vi "niRFUtil FTW Compute AAF Parameter.vi"(10 "Stopband Attenuation (dB)":dbl=85.0 format="%.2f", 11 "Decimation Rate":dbl=1.0) -> (2 "Kaiser Beta":dbl format="%.2f", 3 "AAF Order":i32)   [LabVIEW 2015, in "niRFUtil.lvlib"]
uses:
  niRFUtil.lvlib
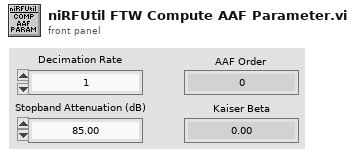
[diagram p1: front panel]
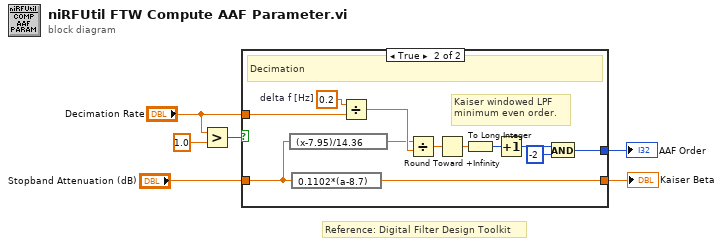
[diagram p0: block diagram]
diagram:
  # "Reference: Digital Filter Design Toolkit"
  n1 = Greater?(x="Decimation Rate", y=1.0) -> (0:w5:bool)
  n2 = case shown="True" w5 {
    tunnel: "Decimation Rate" -> [_ w10]
    tunnel: [_ w9] -> w3
    tunnel: [_ w8] -> w2
    tunnel: "Stopband Attenuation (dB)" -> [_ w7]
    frame False {
    }
    frame True {
      w11 = 0.2  # delta f [Hz]
      # "Kaiser windowed LPF\nminimum even order."
      # "Decimation"
      n3 = expression code="(x-7.95)/14.36"(w7) -> (w15:dbl)
      n4 = expression code="0.1102*(a-8.7)"(w7) -> (w8:dbl)
      n5 = Divide(x=w11, y=w10) -> (x/y=w16:dbl)
      n6 = Divide(x=w15, y=w16) -> (x/y=w12:dbl)
      n7 = Round Toward +Infinity(x=w12) -> (ceil(x): smallest int >= x=w14:dbl)
      n8 = To Long Integer(number=w14) -> (32bit integer=w13:i32)
      n9 = Increment(x=w13) -> (x+1=w17:i32)
      n10 = And(x=w17, y=-2) -> (x .and. y?=w9:i32)
    }
  }
  "AAF Order" <- w3
  "Kaiser Beta" <- w2
